vi "UART_Release.vi"(8 "error in":errorcluster, 11 "instrument handle":refnum<k15>) -> (0 "error out":errorcluster)   [LabVIEW 2024, in "UART.lvlib"]
doc: "Disconnect all the NI PXIe-657x channels and release the hardware"
uses:
  UART.lvlib
  <instrlib>/niDigital/niDigital.llb/niDigital Selected Function.ctl
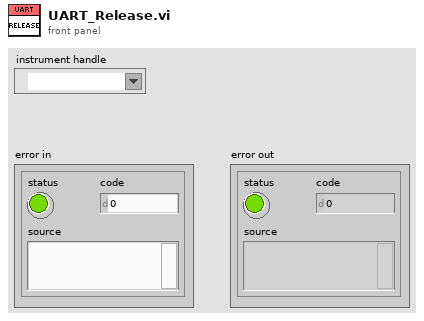
[diagram p1: front panel]
types:
  T1 = typedef "niDigital Selected Function.ctl" = i32
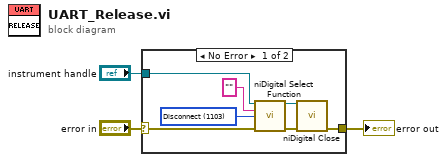
[diagram p0: block diagram]
diagram:
  n1 = case shown="No Error" "error in" {
    selector: "error in" -> [w10 w11]
    tunnel: [w5 w11] -> w2
    tunnel: "instrument handle" -> [w9 _]
    frame No Error {
      w8 = T1 1103 items=["Digital"=1100, "PPMU"=1101, "Off"=1102, "Disconnect"=1103, "RIO"=1104] ("function")
      n2 = call <instrlib>:"niDigital Select Function.vi"("instrument handle"=w9, "channel list"="", "function"=w8, "error in"=w10) -> ("instrument handle out"=w6:refnum<k15>, "error out"=w7:errorcluster)  [unwired: 10 in]
      n3 = call <instrlib>:"niDigital Close.vi"("instrument handle"=w6, "error in"=w7) -> ("error out"=w5:errorcluster)  [unwired: 13 in]
    }
    frame Error {
    }
  }
  "error out" <- w2
